vi "时间锁止.vi"(1 "y":string="2014-10-10") -> ()   [LabVIEW 2013]
panel:
  out "x >= y?":bool
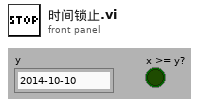
[diagram p1: front panel]
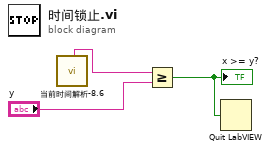
[diagram p0: block diagram]
diagram:
  n1 = call "当前时间解析-8.6.vi"() -> ("日期字符串"=w2:string)  [unwired: 1 in, 18 out]
  n2 = Greater Or Equal?(x=w2, y="y") -> (x >= y?=w3:bool)
  "x >= y?" <- w3
  n3 = Quit LabVIEW(quit? (T)=w3) -> ()
